vi "GraphClusterLogic.vi"(5 "Multimeter":refnum<visa-resource-name>, 7 "Commutator":refnum<visa-resource-name>, 8 "Max. transistor power":dbl=5.0 caption="Max. transistor power [mW]" min=5.0 max=150.0 step=5.0, 9 "Voltage  B":dbl(knob) caption="Voltage B [V]" min=0.0 max=50.0 step=0.01 scale=0.0..50.0 scale format="%#.3f", 10 "Current A":dbl(knob) caption="Current A [mA]" min=0.0 max=50.0 step=0.01 scale=0.0..50.0 scale format="%#.3f", 11 "Power Source":refnum<visa-resource-name>) -> (1 "Ic Array":dbl[](array[numeric]), 2 "Uc Array":dbl[](array[numeric]))   [LabVIEW 2021]
panel:
  out "Uc":dbl
  out "Voltage Array":dbl[](array[numeric])
  out "Trans. power":dbl
  out "Ic":dbl
  out "HP34401":dbl format="%#.3e"
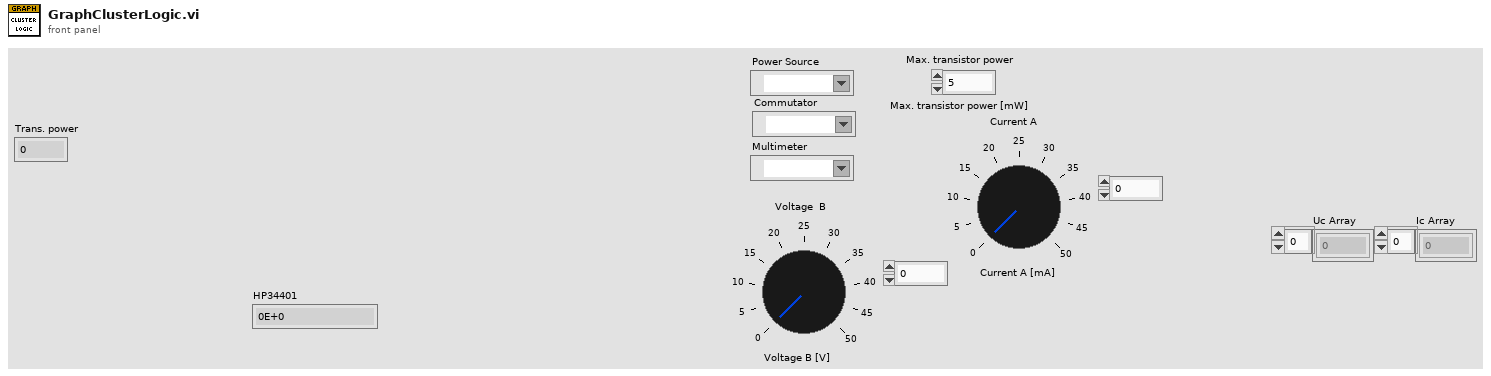
[diagram p1: front panel]
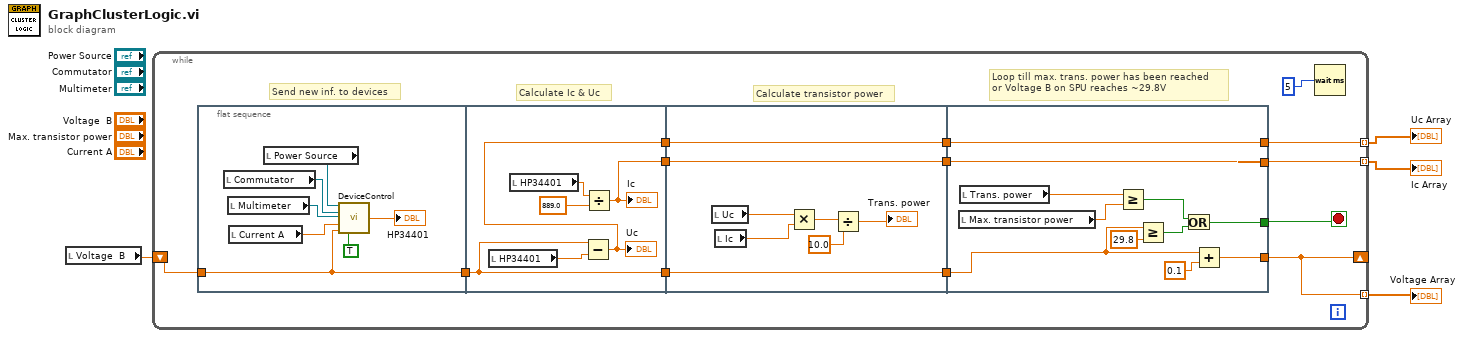
[diagram p0: block diagram]
diagram:
  n1 = local read "Voltage  B"() -> (w4:dbl)
  n2 = while {
    shift-right: [w8] -> _
    shift-left: w4 -> [w15]
    tunnel: [w9] -> w3 mode=indexing
    tunnel: [w8] -> w2 mode=indexing
    tunnel: [w5] -> w1 mode=indexing
    stop <- w16 stop-if-true
    # "Loop till max. trans. power has been reached\nor Voltage B on SPU reaches ~29.8V"
    # "Calculate transistor power"
    # "Calculate Ic & Uc"
    # "Send new inf. to devices"
    n3 = flat-sequence {
      tunnel: w15 -> [w20]
      tunnel: [w20] -> w12
      tunnel: [w27] -> w13
      tunnel: w12 -> [w27]
      tunnel: [w25] -> w11
      tunnel: [w29] -> w7
      tunnel: [w33] -> w14
      tunnel: w13 -> [w33]
      tunnel: w11 -> [w32]
      tunnel: [w32] -> w10
      tunnel: w7 -> [w31]
      tunnel: [w31] -> w6
      tunnel: [w39] -> w16
      tunnel: w14 -> [w43]
      tunnel: [w46] -> w8
      tunnel: w10 -> [w45]
      tunnel: [w45] -> w9
      tunnel: w6 -> [w44]
      tunnel: [w44] -> w5
      frame #0 {
        n4 = local read "Commutator"() -> (w22:refnum<visa-resource-name>)
        n5 = local read "Multimeter"() -> (w21:refnum<visa-resource-name>)
        n6 = local read "Current A"() -> (w18:dbl)
        n7 = local read "Power Source"() -> (w23:refnum<visa-resource-name>)
        n8 = call "DeviceControl.vi"("Power Source"=w23, "Commutator"=w22, "Multimeter"=w21, "Current A"=w18, "Voltage  B"=w20, "PSU A or B"=TRUE) -> ("HP34401"=→"HP34401":dbl)  [unwired: 9 in]
      }
      frame #1 {
        n9 = local read "HP34401"() -> (w26:dbl)
        n10 = local read "HP34401"() -> (w28:dbl)
        n11 = Subtract(x=w27, y=w26) -> (x-y=w25:dbl)
        "Uc" <- w25
        n12 = Divide(x=w28, y=889.0) -> (x/y=w29:dbl)
        "Ic" <- w29
      }
      frame #2 {
        n13 = local read "Uc"() -> (w34:dbl)
        n14 = local read "Ic"() -> (w38:dbl)
        n15 = Multiply(x=w34, y=w38) -> (x*y=w37:dbl)
        n16 = Divide(x=w37, y=10.0) -> (x/y=→"Trans. power":dbl)
      }
      frame #3 {
        n17 = local read "Max. transistor power"() -> (w48:dbl)
        n18 = local read "Trans. power"() -> (w49:dbl)
        n19 = Greater Or Equal?(x=w49, y=w48) -> (x >= y?=w40:bool)
        n20 = Greater Or Equal?(x=w43, y=29.8) -> (x >= y?=w41:bool)
        n21 = Or(x=w40, y=w41) -> (x .or. y?=w39:bool)
        n22 = Add(x=w43, y=0.1) -> (x+y=w46:dbl)
      }
    }
    n23 = Wait (ms)(milliseconds to wait=u32 5) -> ()  [unwired: 1 out]
  }
  "Uc Array" <- w3
  "Voltage Array" <- w2
  "Ic Array" <- w1
